vi "test get all name.vi"() -> ()   [LabVIEW 2018, in "Data Parser.lvclass"]
uses:
  Data Parser.lvclass
panel:
  out "Title Name and Frame Num":cluster{"Name":string, "Num":i32}[](array[cluster])
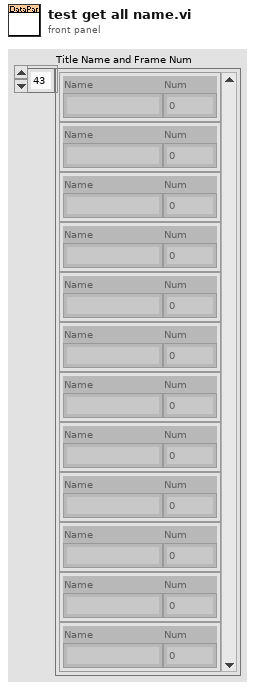
[diagram p1: front panel]
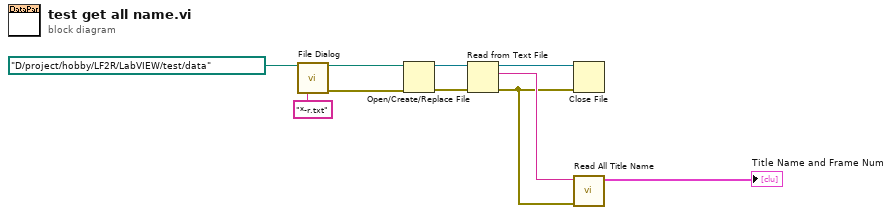
[diagram p0: block diagram]
diagram:
  n1 = call "File Dialog"("start path"=path "D:/project/hobby/LF2R/LabVIEW/test/data", "pattern (all files)"="*-r.txt") -> ("selected path"=w5:path, "error out"=w4:errorcluster)  [unwired: 10 in, 2 out]
  n2 = Open/Create/Replace File(file path (use dialog)=w5, error in=w4) -> (refnum out=w10:refnum<file>, error out=w9:errorcluster)  [unwired: 4 in, 1 out]
  n3 = Read from Text File(file (use dialog)=w10, error in=w9) -> (refnum out=w8:refnum<file>, text=w3:string, error out=w2:errorcluster)  [unwired: 2 in, 1 out]
  n4 = Close File(refnum=w8, error in=w2) -> ()  [unwired: 2 out]
  n5 = call "Read All Title Name.vi"("error in (no error)"=w2, "File String"=w3) -> ("Title Name and Frame Num"=→"Title Name and Frame Num":cluster{"Name":string, "Num":i32}[])  [unwired: 8 in, 1 out]
